vi "Translation.vi"(5 "error in (no error)":errorcluster, 7 "VISA resource name":refnum<visa-resource-name>) -> ()   [LabVIEW 2023]
panel:
  out "error out":errorcluster
  out "return count":u32
  out "read buffer":string
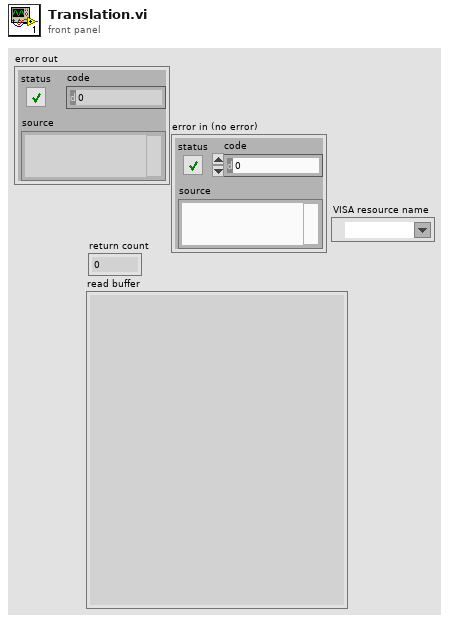
[diagram p1: front panel]
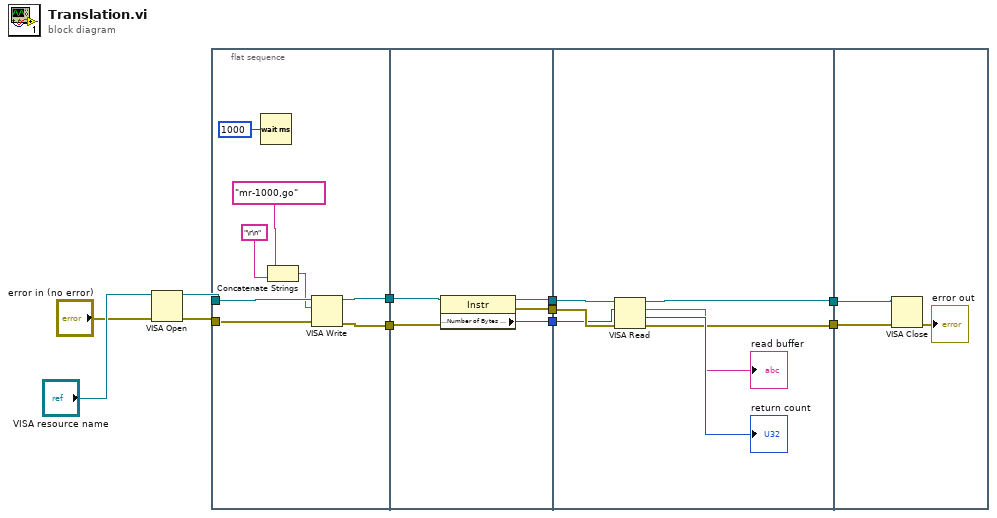
[diagram p0: block diagram]
diagram:
  n1 = VISA Open(error in (no error)="error in (no error)", VISA resource name="VISA resource name") -> (VISA resource name=w3:refnum<visa-resource-name>, error out=w4:errorcluster)  [unwired: 3 in]
  n2 = flat-sequence {
    tunnel: [w17] -> w11
    tunnel: [w16] -> w10
    tunnel: w4 -> [w19]
    tunnel: w3 -> [w18]
    tunnel: w11 -> [w21]
    tunnel: [w22] -> w9
    tunnel: w10 -> [w24]
    tunnel: [w23] -> w8
    tunnel: [w20] -> w7
    tunnel: w9 -> [w31]
    tunnel: w8 -> [w30]
    tunnel: [w27] -> w6
    tunnel: [w26] -> w5
    tunnel: w7 -> [w25]
    tunnel: w6 -> [w34]
    tunnel: w5 -> [w33]
    frame #0 {
      n3 = Wait (ms)(milliseconds to wait=u32 1000) -> ()  [unwired: 1 out]
      n4 = Concatenate Strings("mr-1000,go", "\r\n" ("string")) -> (w13:string)
      n5 = VISA Write(VISA resource name=w18, write buffer=w13, error in (no error)=w19) -> (VISA resource name out=w16:refnum<visa-resource-name>, error out=w17:errorcluster)  [unwired: 1 out]
    }
    frame #1 {
      n6 = property class="Instr"(reference=w24, error in=w21) -> (reference out=w23:refnum<visa-resource-name>, error out=w22:errorcluster, "Serial Settings:Number of Bytes at Serial Port"=w20:u32)
    }
    frame #2 {
      n7 = VISA Read(VISA resource name=w30, byte count=w25, error in (no error)=w31) -> (VISA resource name out=w27:refnum<visa-resource-name>, read buffer=→"read buffer":string, return count=→"return count":u32, error out=w26:errorcluster)
    }
    frame #3 {
      n8 = VISA Close(VISA resource name=w34, error in (no error)=w33) -> (error out=→"error out":errorcluster)
    }
  }
